vi "ControlMainGUIWindow.vi"(8 "ErrorIn":errorcluster, 10 "ShowProcessWindow":bool, 11 "ReferenceIn":refnum<class "TraceWindow.lvclass">) -> (0 "ErrorOut":errorcluster, 2 "Dummy":bool, 3 "ReferenceOut":refnum<class "TraceWindow.lvclass">)   [LabVIEW 2021, in "TraceWindow.lvlib" / "TraceWindow.lvclass"]
uses:
  TraceWindow.lvclass
  protected/TraceWindow_MessageData.ctl
  9f903c85-2847-4db9-ba05-d8e85b2316fc.vi
  protected/MainGUIRepository.vi
  TraceWindow.lvclass/TraceWindow.ctl
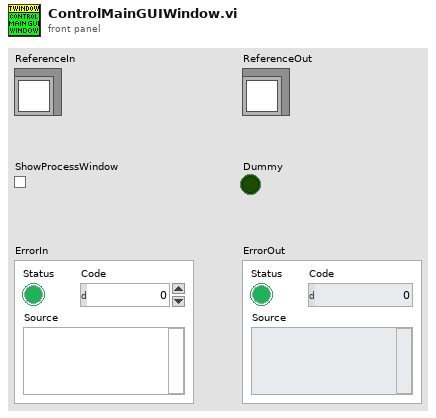
[diagram p1: front panel]
types:
  T1 = typedef "TraceWindow.lvlib/TraceWindow.lvclass/TraceWindow_MessageData.ctl" = cluster{"Show":cluster{"Send":cluster{"State":bool}, "Receive":cluster{"Dummy":bool}}, "WriteTraceQueue":cluster{"Send":cluster{"TraceQueue":refnum<queue>}, "Receive":cluster{"Dummy":bool}}}
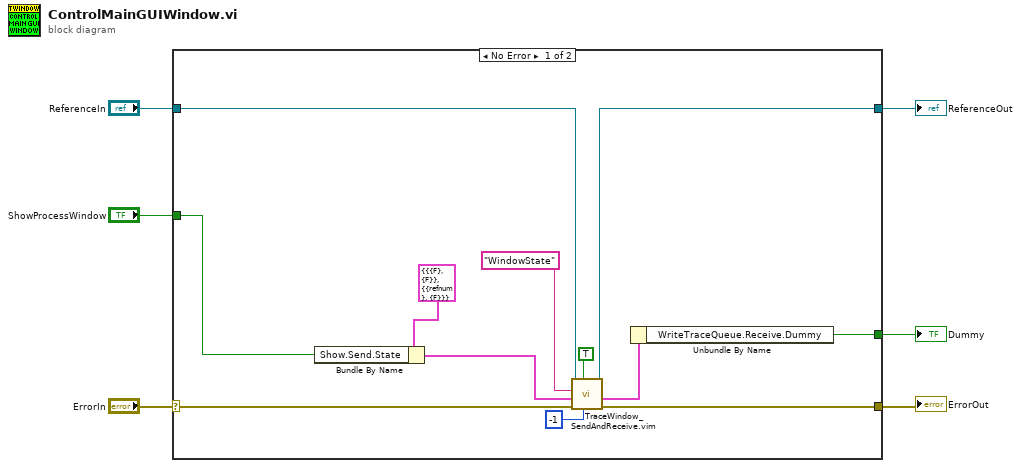
[diagram p0: block diagram]
diagram:
  n1 = case shown="No Error" "ErrorIn" {
    selector: "ErrorIn" -> [w18 w20]
    tunnel: [w17 w20] -> w5
    tunnel: [w14 w19] -> w3
    tunnel: "ReferenceIn" -> [w15 w19]
    tunnel: "ShowProcessWindow" -> [w12 _]
    tunnel: [w9 _] -> w1
    frame No Error {
      n2 = Bundle By Name(cluster=T1 {"Show"={"Send"={"State"=FALSE}, "Receive"={"Dummy"=FALSE}}, "WriteTraceQueue"={"Send"={"TraceQueue"=refnum}, "Receive"={"Dummy"=FALSE}}} ("MessageData"), "Show.Send.State"=w12) -> (w11:T1)
      n3 = call "TraceWindow_SendAndReceive.vim"("TimeoutInMs(-1)"=-1 ("timeout in ms (-1)"), "ShouldWeWaitForResponse"=TRUE, "ErrorIn"=w18, "Data"=w11, "Command"="WindowState", "ReferenceIn"=w15) -> ("ErrorOut"=w17:errorcluster, "ReplyData"=w10:T1, "ReferenceOut"=w14:refnum<class "TraceWindow.lvclass">)  [unwired: 3 in]
      n4 = Unbundle By Name(w10) -> ("WriteTraceQueue.Receive.Dummy"=w9:bool)
    }
    frame Error {
    }
  }
  "ErrorOut" <- w5
  "ReferenceOut" <- w3
  "Dummy" <- w1
